vi "Match Pattern Demo RasPi Camera.vi"() -> ()   [LabVIEW 2014]
uses:
  vi.lib/Q-WaveSystems/QwaveSys Raspberry Pi for LabVIEW Home-Education/QwaveSys Raspberry Pi Library.lvlib
panel:
  out "yB":i32
  out "yT":i32
  out "xR":i32
  out "xL":i32
  in  "Cmd":string(combo)="raspistill -t 1 -md 6 -o cam.jpg -w 640 -h 480"
  out "standard error":string
  out "standard output":string
  out "score":dbl=1.0
  out "2D Picture":picture
  out "Template":picture
  out "Output":picture
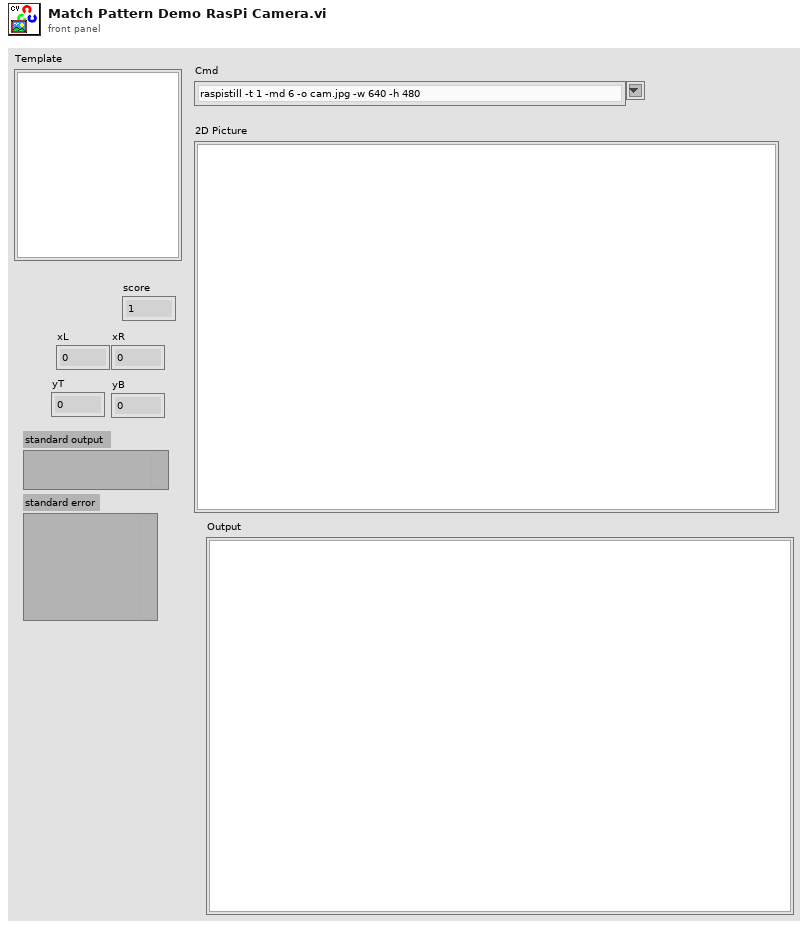
[diagram p1: front panel]
types:
  T1 = typedef "imagedata.ctl" = cluster{"image type":i32, "image depth":i32, "image":u8[], "mask":u8[], "colors":u32[], "Rectangle":cluster{"left":i16, "top":i16, "right":i16, "bottom":i16}}
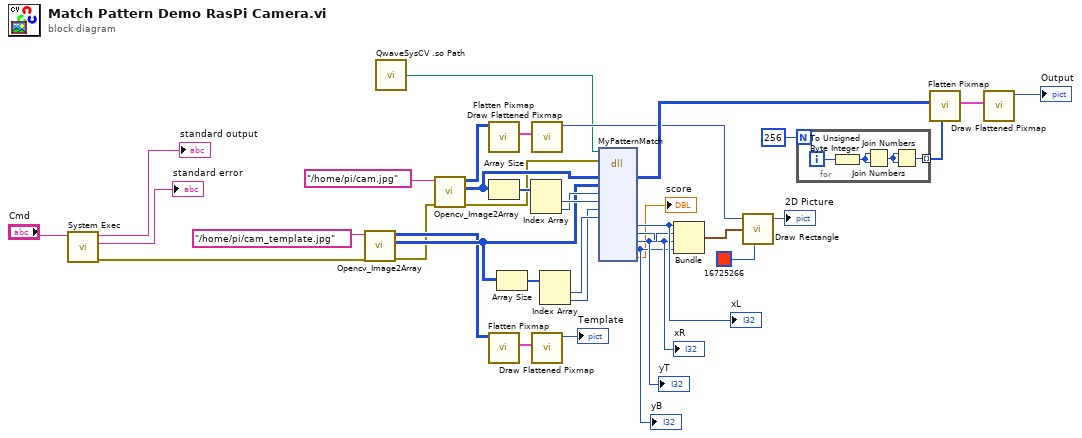
[diagram p0: block diagram]
diagram:
  n1 = call <vilib>:"System Exec.vi"("command line"="Cmd") -> ("error out"=w5:errorcluster, "standard error"=→"standard error":string, "standard output"=→"standard output":string)  [unwired: 7 in, 1 out]
  n2 = call "Opencv_Image2Array.vi"("error in (no error)"=w5, "filename"="/home/pi/cam_template.jpg") -> ("error out"=w4:errorcluster, "Image Pixels Gray"=w29:u8[][], "Image Pixels 24 bits"=w22:u32[][])  [unwired: 7 in]
  n3 = call "QwaveSysCV .so Path.vi"() -> ("QwaveSys .so Path"=w1:path)  [unwired: 5 in]
  n4 = call "Opencv_Image2Array.vi"("error in (no error)"=w4, "filename"="/home/pi/cam.jpg") -> ("error out"=w3:errorcluster, "Image Pixels Gray"=w30:u8[][], "Image Pixels 24 bits"=w17:u32[][])  [unwired: 7 in]
  n5 = call <vilib>:"Flatten Pixmap.vi"("24-bit pixmap"=w17) -> ("image data"=w18:T1)  [unwired: 10 in]
  n6 = Array Size(array=w30) -> (size(s)=w36:i32[])
  n7 = call <vilib>:"Flatten Pixmap.vi"("24-bit pixmap"=w22) -> ("image data"=w24:T1)  [unwired: 10 in]
  n8 = Array Size(array=w29) -> (size(s)=w33:i32[])
  n9 = Index Array(array=w36) -> (element #1=w35:i32, element #2=w34:i32)  [unwired: 2 in]
  n10 = call <vilib>:"Draw Flattened Pixmap.vi"("image data"=w18) -> ("new picture"=w10:picture)  [unwired: 8 in]
  n11 = call <vilib>:"Draw Flattened Pixmap.vi"("image data"=w24) -> ("new picture"=→"Template":picture)  [unwired: 8 in]
  n12 = Index Array(array=w33) -> (element #1=w32:i32, element #2=w31:i32)  [unwired: 2 in]
  n13 = dll-call lib="libqwavesys.so" fn="MyPatternMatch"(path in=w1, error in=w3, "src"=w30, "templ"=w29, "src_cols"=w34, "src_rows"=w35, "templ_cols"=w31, "templ_rows"=w32) -> ("src"=w20:u8[][], "xL"=w15:i32, "xR"=w13:i32, "yT"=w14:i32, "yB"=w12:i32, "score"=→"score":dbl)  [unwired: 12 in, 2 out]
  "xL" <- w15
  "xR" <- w13
  "yT" <- w14
  "yB" <- w12
  n14 = Bundle("xL"=w15, "yT"=w14, "xR"=w13, "yB"=w12) -> (w16:cluster{"xL":i32, "yT":i32, "xR":i32, "yB":i32})  [unwired: 1 in]
  n15 = call <vilib>:"Draw Rectangle.vi"("picture"=w10, "rect"=w16, "color(black)"=u32 16725266) -> ("new picture"=→"2D Picture":picture)  [unwired: 6 in]
  n16 = for {
    N: 256 -> [_]
    tunnel: [w40] -> w19 mode=indexing
    i -> [w38]
    n17 = To Unsigned Byte Integer(number=w38) -> (unsigned 8bit integer=w37:u8)
    n18 = Join Numbers(hi=w37, lo=w37) -> ((hi.lo)=w39:u16)
    n19 = Join Numbers(hi=w39, lo=w39) -> ((hi.lo)=w40:u32)
  }
  n20 = call <vilib>:"Flatten Pixmap.vi"("colors"=w19, "8-bit pixmap"=w20) -> ("image data"=w26:T1)  [unwired: 9 in]
  n21 = call <vilib>:"Draw Flattened Pixmap.vi"("image data"=w26) -> ("new picture"=→"Output":picture)  [unwired: 8 in]
